vi "Throttle.vi"(9 "request data":bool=TRUE, 11 "throttle":u16) -> (1 "throttled request":bool)   [LabVIEW 2023, in "Aurora64b66b Utilities FPGA.lvlib"]
uses:
  Aurora64b66b Utilities FPGA.lvlib
  Program Files/NI/LVAddons/niidl/1/instr.lib/_niInstr/Basic Elements/v1/FPGA/niInstr Basic Elements v1 FPGA.lvlib
  Program Files/NI/LVAddons/niidl/1/instr.lib/_niInstr/Basic Elements/v1/FPGA/Private/Count Up U16.vi
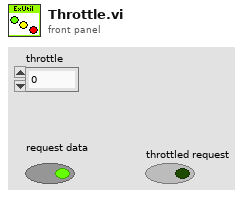
[diagram p1: front panel]
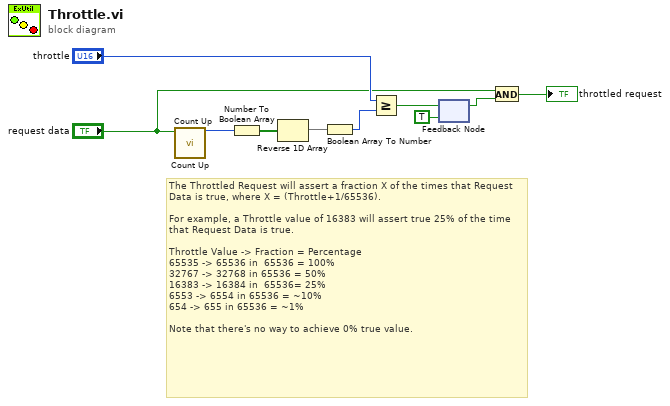
[diagram p0: block diagram]
diagram:
  # "The Throttled Request will assert a fraction X of the times that Request Data is true, where X = (Throttle+1/65536).\n\nFor example, a Throttle value of 16383 will assert true 25% of the time that Request Data is true.\n\nThrottle Value -> Fraction = Percentage\n65535 -> 65536 in  65536 = 100%\n32767 -> 32768 in 65536 = 50%\n16383 -> 16384 in  65536= 25%\n6553 -> 6554 in 65536 = ~10%\n654 -> 655 in 65536 = ~1%\n\nNote that there's no way to achieve 0% true value."
  n1 = call-poly "Count Up.vi"() -> ()  [unwired: 15 in, 1 out]
  n2 = call-poly "Count Up.vi"("increment"="request data") -> ("count out"=w10:u16)  [unwired: 14 in]
  n3 = Number To Boolean Array(number=w10) -> (Boolean array=w9:bool[])
  n4 = Reverse 1D Array(array=w9) -> (reversed array=w8:bool[])
  n5 = Boolean Array To Number(Boolean array=w8) -> (number=w7:u16)
  n6 = Greater Or Equal?(x="throttle", y=w7) -> (x >= y?=w6:bool)
  n7 = feedback #1(TRUE) -> (w5:bool)
  n8 = feedback-in #1(w6) -> ()
  n9 = And(x="request data", y=w5) -> (x .and. y?=→"throttled request":bool)
